vi "Property Tree_Remove empty display-only parents.vi"(7 "Action":T1, 10 "Disabled?":bool[](array[boolean]), 11 "Tree Arr":T2(array[cluster])) -> (2 "Disabled? Out":bool[](array[boolean]), 3 "Tree Arr Out":T2(array[cluster]))   [LabVIEW 2023]
doc: "If item is disabled and it has the same indent level as the next item in the array, then it can be removed, as it has no decendants to display\n\nAlso deal with redundant dividers. (first, last, and repeated, which can happen when filtering)"
uses:
  controls/action enum.ctl
  <userlib>/_OpenG.lib/array/array.llb/Remove Duplicates from 1D Array (I32)__ogtk.vi
  <userlib>/_OpenG.lib/array/array.llb/openg_array.lvlib
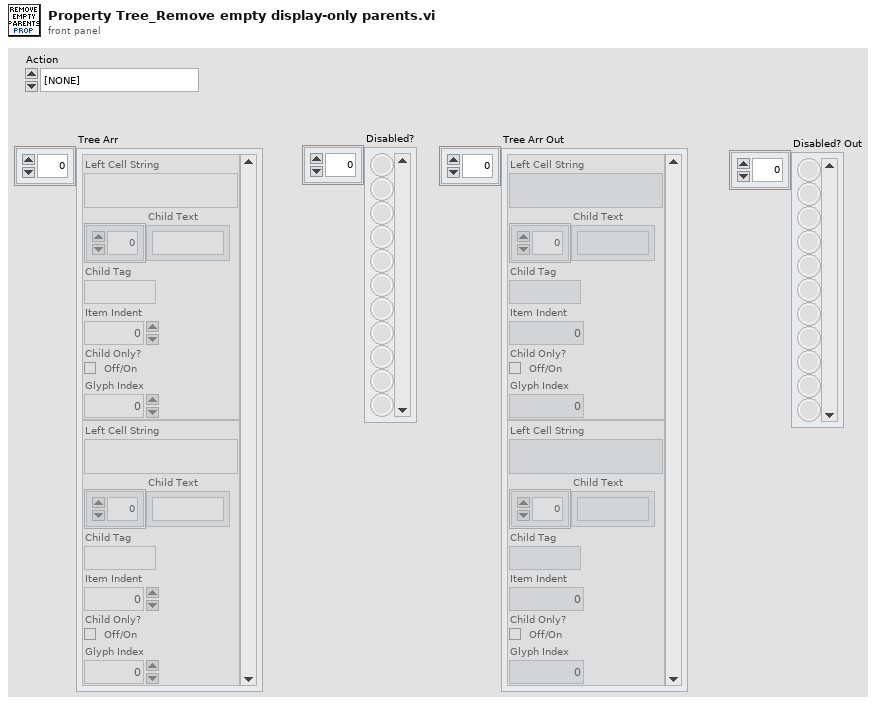
[diagram p1: front panel]
types:
  T1 = typedef "action enum.ctl" = enum16{"[NONE]", "APP_SEPARATOR", "Wire Bundle", "Wire Unbundle", "Terminal Unbundle", "Terminal Bundle", "Bundler Move Up", "Bundler Move Down", "Bundler Insert", "Bundler Remove", "Bundler Remove Unwired", "Bundler Reorder", "In Place Insert", "In Place Remove", "In Place Remove Unwired", "In Place Reorder", "Wire Properties", "Wire Method", "Terminal Properties", "Terminal Method", "Property Move Up", "Property Move Down", "Properties Insert", "Properties Remove", "Properties Remove Unwired", "Properties Reorder", "Method Change", "Class For Constant", "Class For Control", "Class For Node", "Class Name to Clipboard"}
  T2 = cluster{"Left Cell String":string, "Child Text":string[], "Child Tag":string, "Item Indent":i32, "Child Only?":bool, "Glyph Index":i32}[]
  T3 = enum16{"Unknown", "Base", "Scripting", "Private", "Deprecated", "None", "Divider"}
  T4 = cluster{"Left Cell String":string, "Child Text":string[], "Child Tag":string, "Item Indent":i32, "Child Only?":bool, "Glyph Index":i32}
  T5 = cluster{"Index":u16, "Property Type":enum16{"Unknown", "Base", "Scripting", "Private", "Deprecated", "None", "Divider"}, "ID String":string, "Dotted ID String":string, "Class":string, "Parent":string, "Display name full":string, "Display name short":string, "Parents Array":string[], "Indent":u16}
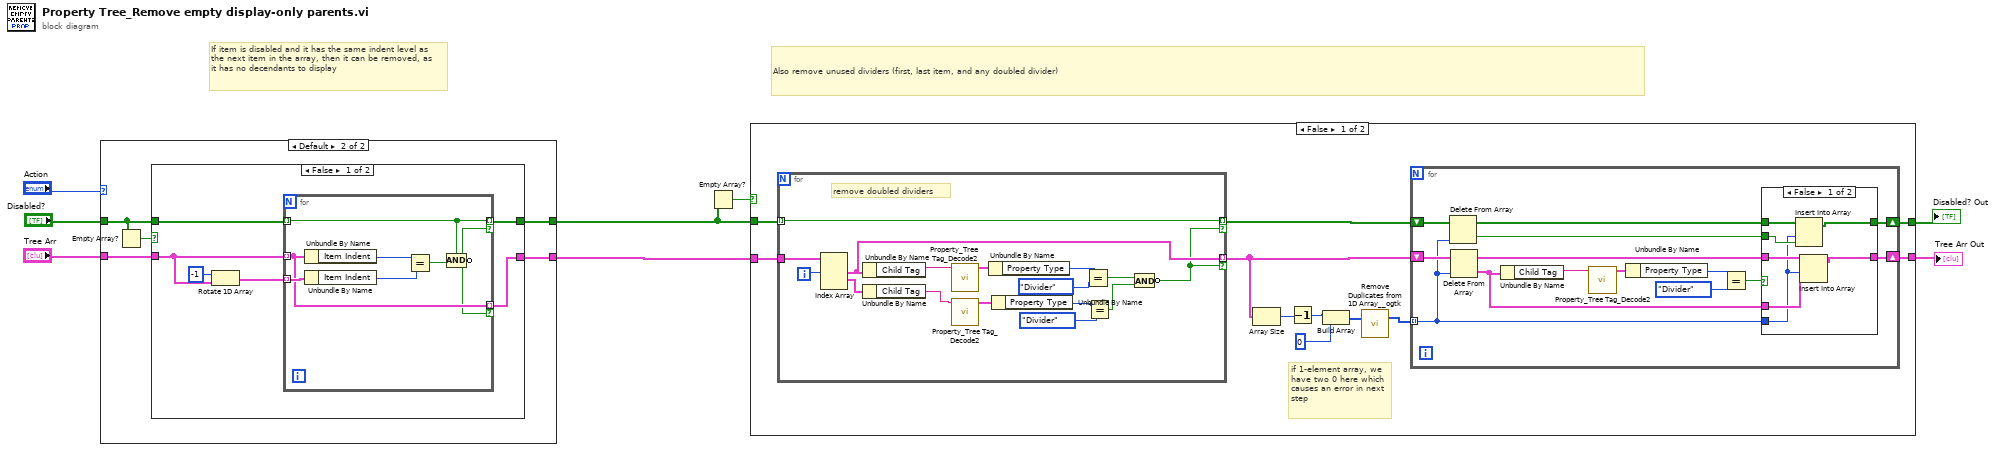
[diagram p0: block diagram]
diagram:
  # "Also remove unused dividers (first, last item, and any doubled divider)"
  # "If item is disabled and it has the same indent level as the next item in the array, then it can be removed, as it has no decendants to display"
  n1 = case shown="Default" "Action" {
    tunnel: "Tree Arr" -> [w9 w15]
    tunnel: "Disabled?" -> [w10 w11]
    tunnel: [w9 w14] -> w5
    tunnel: [w10 w13] -> w2
    frame "Properties Remove", "Properties Reorder" {
    }
    frame Default {
      n2 = Empty Array?(array=w11) -> (empty?=w12:bool)
      n3 = case shown="False" w12 {
        tunnel: w15 -> [w21 w29]
        tunnel: w11 -> [w19 w30]
        tunnel: [w18 w29] -> w14
        tunnel: [w16 w30] -> w13
        frame False {
          n4 = Rotate 1D Array(1:w21, 2:-1 ("n")) -> (0:w20:T2)
          n5 = for {
            tunnel: w21 -> [w24] mode=indexing
            tunnel: w20 -> [w25] mode=indexing
            tunnel: w19 -> [w23] mode=indexing
            tunnel: [w24] -> w18 mode=indexing if=w22
            tunnel: [w23] -> w16 mode=indexing if=w22
            n6 = Unbundle By Name(w24) -> ("Item Indent"=w28:i32)
            n7 = Unbundle By Name(w25) -> ("Item Indent"=w27:i32)
            n8 = Equal?(x=w28, y=w27) -> (x = y?=w26:bool)
            n9 = Compound Arithmetic op=AND(w23, w26) -> (invert w22:bool)
          }
        }
        frame True {
        }
      }
    }
  }
  n10 = Empty Array?(array=w2) -> (empty?=w1:bool)
  n11 = case shown="False" w1 {
    tunnel: w2 -> [w41 w82]
    tunnel: w5 -> [w40 w81]
    tunnel: [w33 w81] -> w4
    tunnel: [w32 w82] -> w3
    frame False {
      # "if 1-element array, we have two 0 here which causes an error in next step"
      n12 = for {
        tunnel: w40 -> [w68]
        tunnel: w41 -> [w70] mode=indexing
        tunnel: [w69] -> w37 mode=indexing if=w65
        tunnel: [w70] -> w36 mode=indexing if=w65
        i -> [w67]
        # "remove doubled dividers"
        n13 = Index Array(array=w68, index #1=w67) -> (element #1=w69:T4, element #2=w80:T4)  [unwired: 2 in, 1 out]
        n14 = Unbundle By Name(w69) -> ("Child Tag"=w79:string)
        n15 = Unbundle By Name(w80) -> ("Child Tag"=w78:string)
        n16 = call "Property_Tree Tag_Decode2.vi"("Tag In"=w79) -> ("TagData"=w77:T5)  [unwired: 10 in]
        n17 = call "Property_Tree Tag_Decode2.vi"("Tag In"=w78) -> ("TagData"=w76:T5)  [unwired: 10 in]
        n18 = Unbundle By Name(w77) -> ("Property Type"=w75:T3)
        n19 = Unbundle By Name(w76) -> ("Property Type"=w73:T3)
        n20 = Equal?(x=w75, y=T3."Divider" ("Property Type")) -> (x = y?=w66:bool)
        n21 = Equal?(x=w73, y=T3."Divider" ("Property Type")) -> (x = y?=w71:bool)
        n22 = Compound Arithmetic op=AND(w66, w71) -> (invert w65:bool)
      }
      n23 = Array Size(array=w37) -> (size(s)=w39:i32)
      n24 = Decrement(x=w39) -> (x-1=w38:i32)
      n25 = Build Array(w38, 0 ("element")) -> (w35:i32[])
      n26 = call-poly <userlib>:"Remove Duplicates from 1D Array__ogtk.vi"("Input Array"=w35) -> ("Output Array"=w31:i32[])  [unwired: 1 out]
      n27 = for {
        tunnel: w31 -> [w43] mode=indexing
        shift-right: [w46] -> w33
        shift-left: w37 -> [w51]
        shift-right: [w48] -> w32
        shift-left: w36 -> [w52]
        n28 = Delete From Array(array=w52, index=w43) -> (deleted portion=w44:bool, array with subset deleted=w47:bool[])  [unwired: 1 in]
        n29 = Delete From Array(array=w51, index=w43) -> (deleted portion=w42:T4, array with subset deleted=w45:T2)  [unwired: 1 in]
        n30 = Unbundle By Name(w42) -> ("Child Tag"=w53:string)
        n31 = call "Property_Tree Tag_Decode2.vi"("Tag In"=w53) -> ("TagData"=w54:T5)  [unwired: 10 in]
        n32 = Unbundle By Name(w54) -> ("Property Type"=w55:T3)
        n33 = Equal?(x=w55, y=T3."Divider" ("Property Type")) -> (x = y?=w49:bool)
        n34 = case shown="False" w49 {
          tunnel: [w60 w64] -> w48
          tunnel: w47 -> [w62 w64]
          tunnel: [w57 w63] -> w46
          tunnel: w45 -> [w58 w63]
          tunnel: w44 -> [w61 _]
          tunnel: w43 -> [w56 _]
          tunnel: w42 -> [w59 _]
          frame False {
            n35 = Insert Into Array(array=w62, index=w56, new element=w61) -> (w60:bool[])
            n36 = Insert Into Array(array=w58, index=w56, new element=w59) -> (w57:T2)
          }
          frame True {
          }
        }
      }
    }
    frame True {
    }
  }
  "Tree Arr Out" <- w4
  "Disabled? Out" <- w3
